vi "Build Queue Data.vi"(8 "error in (no error)":errorcluster, 11 "Data from FIFO":u64[](array[numeric])) -> (0 "error out":errorcluster, 3 "Data to Queue":T1[](array[typedef]))   [LabVIEW 2016]
uses:
  Typedefs/Monitor Data Element.ctl
  Typedefs/Monitor Data Operation.ctl
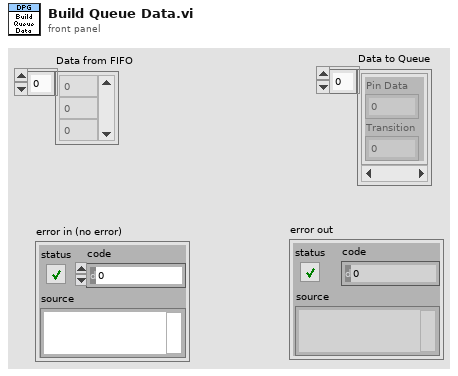
[diagram p1: front panel]
types:
  T1 = typedef "Monitor Data Element.ctl" = cluster{"Pin Data":u32, "Transition ":u32}
  T2 = typedef "Monitor Data Operation.ctl" = enum16{"Obtain", "Enqueue", "Read Elements", "Flush", "Release", "Read Last Element"}
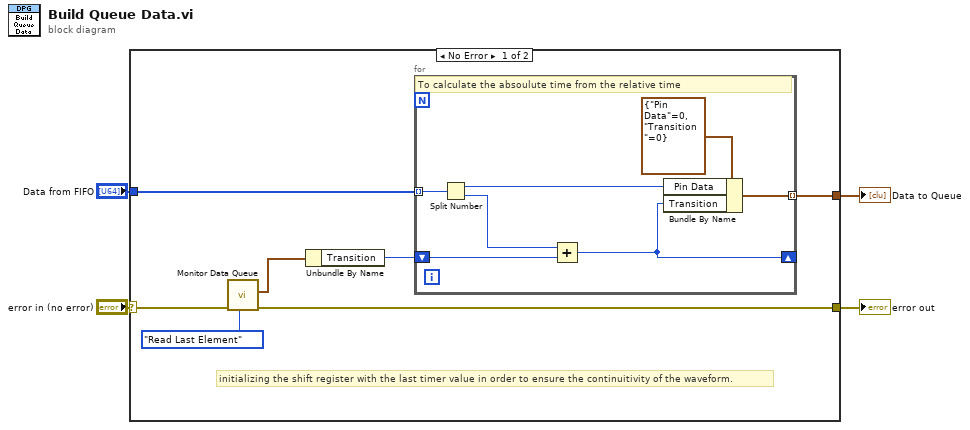
[diagram p0: block diagram]
diagram:
  n1 = case shown="No Error" "error in (no error)" {
    selector: "error in (no error)" -> [w5 w19]
    tunnel: "Data from FIFO" -> [w11 _]
    tunnel: [w8 w19] -> w2
    tunnel: [w9 _] -> w1
    frame No Error {
      # "initializing the shift register with the last timer value in order to ensure the continuitivity of the waveform."
      n2 = call "Monitor Data Queue.vi"("Queue Function"=Monitor_Data_Operation."Read Last Element", "error in (no error)"=w5) -> ("error out"=w8:errorcluster, "Last Queue Element"=w7:T1)  [unwired: 6 in, 2 out]
      n3 = Unbundle By Name(w7) -> ("Transition"=w10:u32)
      n4 = for {
        tunnel: w11 -> [w18] mode=indexing
        shift-right: [w14] -> _
        shift-left: w10 -> [w17]
        tunnel: [w13] -> w9 mode=indexing
        # "To calculate the absoulute time from the relative time"
        n5 = Split Number(x=w18) -> (hi(x)=w15:u32, lo(x)=w12:u32)
        n6 = Add(x=w12, y=w17) -> (x+y=w14:u32)
        n7 = Bundle By Name(cluster=T1 {"Pin Data"=0, "Transition "=0} ("Monitor Data Element"), "Pin Data"=w15, "Transition"=w14) -> (w13:T1)
      }
    }
    frame Error {
    }
  }
  "error out" <- w2
  "Data to Queue" <- w1
